vi "Get Arbitrary Waveform Info.vi"(7 "Attribute Name (0: Average)":i32(ring) items=["Average", "Crest Factor", "Points Count", "Peak-To-Peak Value"], 8 "error in (no error)":errorcluster, 9 "Arbitrary Waveform Name (ARB1)":string="ARB1", 10 "Channel (1:1)":i32(ring)=1 items=["1"=1, "2"=2], 11 "VISA resource name":refnum<visa-resource-name>) -> (0 "error out":errorcluster, 2 "Attribute Value":dbl, 3 "VISA resource name out":refnum<visa-resource-name>)   [LabVIEW 2023, in "Keysight-33500B.lvlib"]
doc: "Returns the geometry property like arithmetic average, crest factor, points count or peak-to-peak value of specified waveform.\n\n<b>Note</b>:\n(1) This VI does not check the instrument status."
uses:
  Keysight-33500B.lvlib
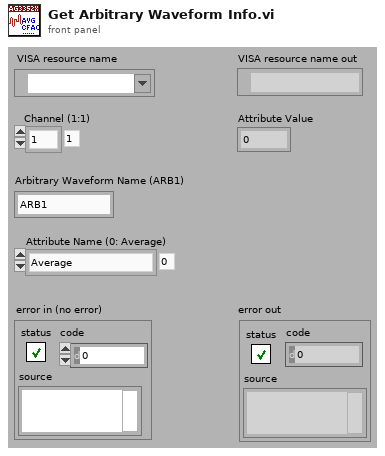
[diagram p1: front panel]
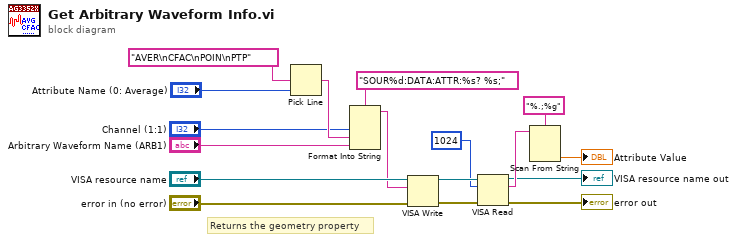
[diagram p0: block diagram]
diagram:
  # "Returns the geometry property"
  n1 = Pick Line(multi-line string="AVER\nCFAC\nPOIN\nPTP", line index="Attribute Name (0: Average)") -> (output string=w9:string)  [unwired: 1 out]
  n2 = Format Into String(format string="SOUR%d:DATA:ATTR:%s? %s;", "Channel (1:1)", w9, "Arbitrary Waveform Name (ARB1)") -> (resulting string=w7:string)  [unwired: 2 in, 1 out]
  n3 = VISA Write(VISA resource name="VISA resource name", write buffer=w7, error in (no error)="error in (no error)") -> (VISA resource name out=w15:refnum<visa-resource-name>, error out=w14:errorcluster)  [unwired: 1 out]
  n4 = VISA Read(VISA resource name=w15, byte count=u32 1024, error in (no error)=w14) -> (VISA resource name out=→"VISA resource name out":refnum<visa-resource-name>, read buffer=w5:string, error out=→"error out":errorcluster)  [unwired: 1 out]
  n5 = Scan From String(format string="%.;%g", input string=w5) -> (output 1=→"Attribute Value":dbl)  [unwired: 2 in, 4 out]
